vi "RD Analog In Trigger Condition Set.vi"(8 "error in (no error)":errorcluster caption="错误输入（无错误）", 10 "trigcond":enum16{"Raising", "Falling", "Either"}(ring), 11 "handle":u64) -> (0 "error out":errorcluster caption="错误输出", 2 "function return":i32, 3 "handle out":u64)   [LabVIEW 2018, in "InstrumentsPlayground.lvlib"]
doc: "CLIFFAPI int CliffAnalogInTriggerConditionSet(FT_HANDLE handle, CLIFFTriggerSlope trigcond);\nCLIFFTriggerSlope: 0 raising ; 1 falling ; 2 either."
uses:
  InstrumentsPlayground.lvlib
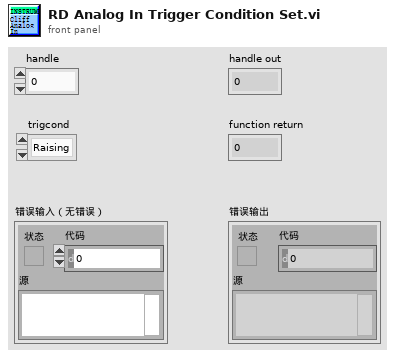
[diagram p1: front panel]
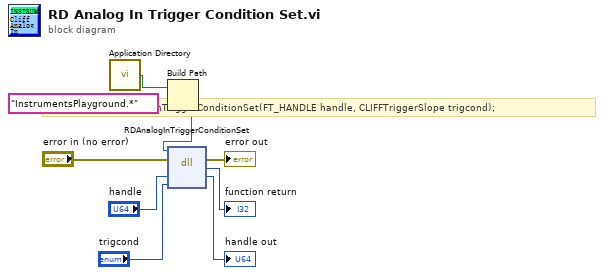
[diagram p0: block diagram]
diagram:
  # "CLIFFAPI int CliffAnalogInTriggerConditionSet(FT_HANDLE handle, CLIFFTriggerSlope trigcond);"
  n1 = call <vilib>:"Application Directory.vi"() -> ("Application Directory"=w2:path)
  n2 = Build Path(base path=w2, name or relative path="InstrumentsPlayground.*" ("名称或相对路径")) -> (appended path=w1:path)
  n3 = dll-call lib="E:/work/YZCourse_Xtext/Cliff/API/LabVIEW lib/InstrumentsPlayground.*" fn="RDAnalogInTriggerConditionSet"(path in=w1, error in="error in (no error)", "handle"="handle", "trigcond"="trigcond") -> (error out=→"error out":errorcluster, "返回类型"=→"function return":i32, "handle"=→"handle out":u32)  [unwired: 2 in, 1 out]
